vi "JTMonitor.vi"() -> ()   [LabVIEW 2016]
uses:
  Global/Global Variables/Data_Display_global.vi
panel:
  out "P5":dbl format="%#_13g"
  out "P3":dbl format="%#_13g"
  out "P2":dbl format="%#_13g"
  out "P1":dbl format="%#_13g"
  out "Comp":bool=TRUE
  out "FP":bool=TRUE
  out "V9":bool=TRUE
  out "V5":bool=TRUE
  out "V4":bool=TRUE
  out "V2":bool=TRUE
  out "V1":bool=TRUE
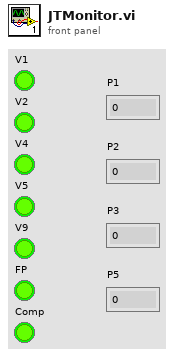
[diagram p1: front panel]
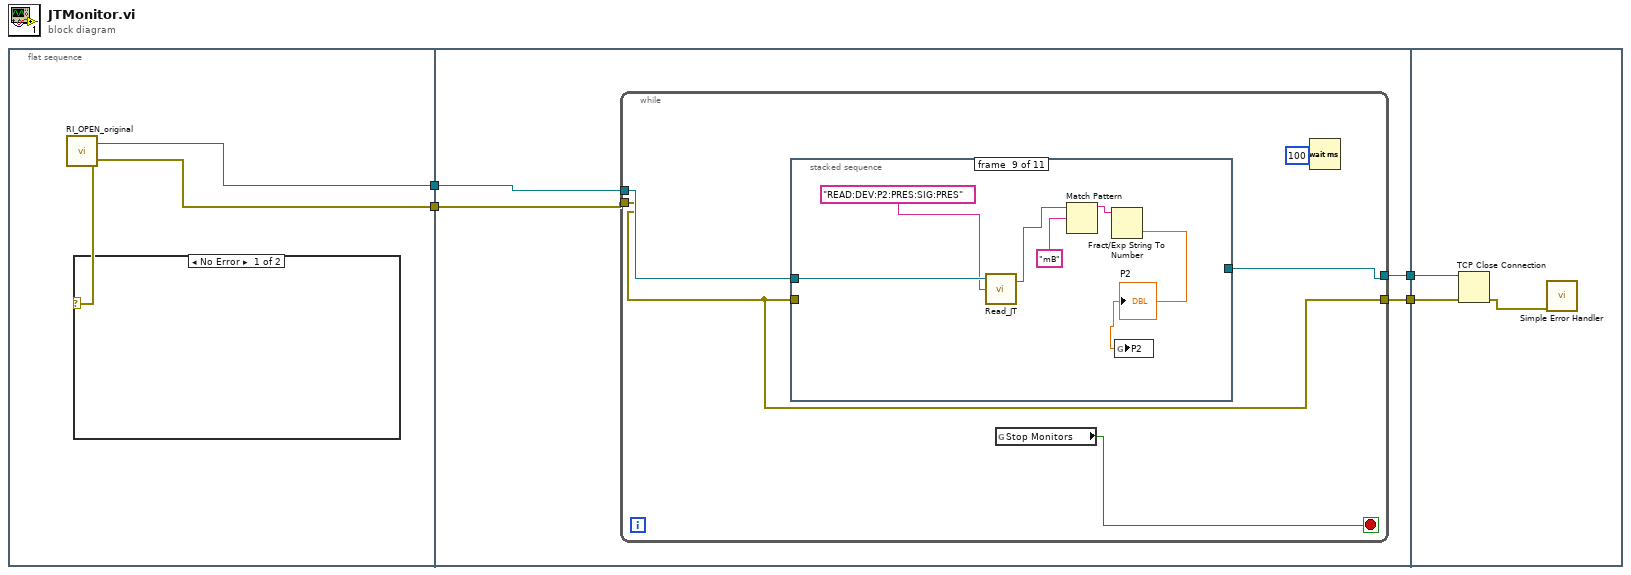
[diagram p0: block diagram]
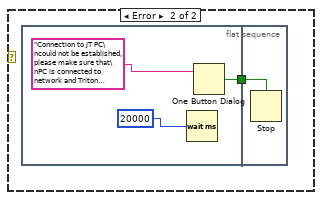
[diagram p2: hidden frame]
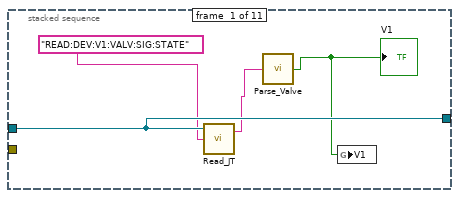
[diagram p3: hidden frame]
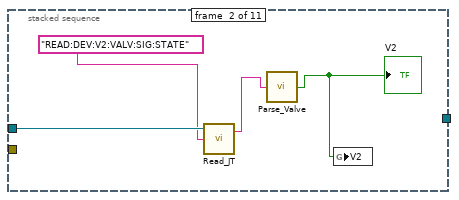
[diagram p4: hidden frame]
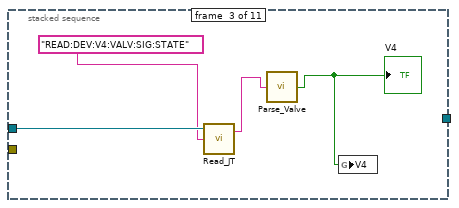
[diagram p5: hidden frame]
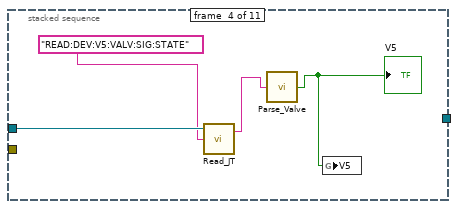
[diagram p6: hidden frame]
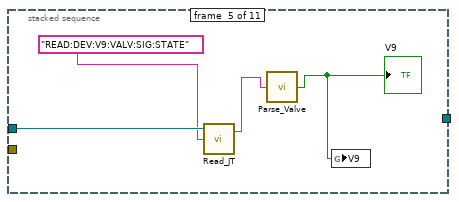
[diagram p7: hidden frame]
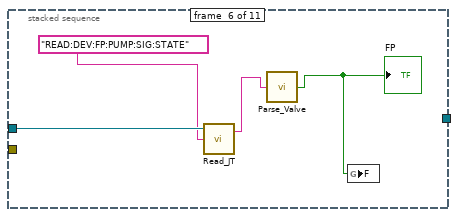
[diagram p8: hidden frame]
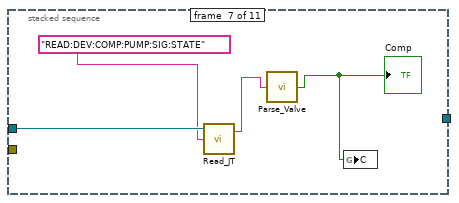
[diagram p9: hidden frame]
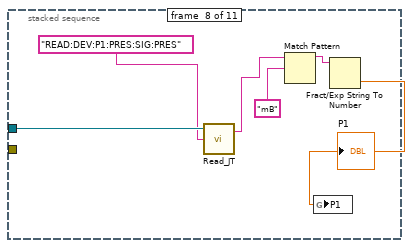
[diagram p10: hidden frame]
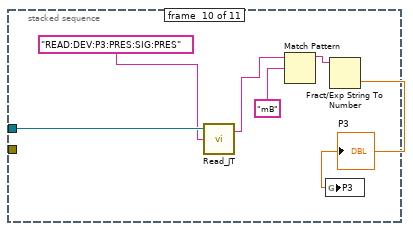
[diagram p11: hidden frame]
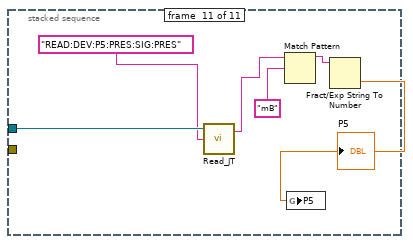
[diagram p12: hidden frame]
diagram:
  n1 = flat-sequence {
    tunnel: [w6] -> w2
    tunnel: [w5] -> w1
    tunnel: [w15] -> w4
    tunnel: [w14] -> w3
    tunnel: w2 -> [w13]
    tunnel: w1 -> [w12]
    tunnel: w4 -> [w74]
    tunnel: w3 -> [w73]
    frame #0 {
      n2 = call "RI_OPEN_original.vi"() -> ("error out"=w5:errorcluster, "connection ID"=w6:refnum<k5>)  [unwired: 3 in]
      n3 = case shown="No Error" w5 {
        frame No Error {
        }
        frame Error {
          n4 = flat-sequence {
            tunnel: [w8] -> w7
            tunnel: w7 -> [w11]
            frame #0 {
              n5 = Wait (ms)(milliseconds to wait=20000) -> ()  [unwired: 1 out]
              n6 = One Button Dialog(message="Connection to JT PC\ncould not be established, please make sure that\nPC is connected to network and Triton control software is running.\n\nThe JT monitor will be restarted in 20 seconds if the status monitor is not stopped meanwhile") -> (true=w8:bool)  [unwired: 1 in]
            }
            frame #1 {
              n7 = Stop(stop? (T)=w11) -> ()
            }
          }
        }
      }
    }
    frame #1 {
      n8 = while {
        tunnel: w13 -> [w19]
        tunnel: w12 -> [w17]
        tunnel: [w18] -> w15
        tunnel: [w17] -> w14
        stop <- w20 stop-if-true
        n9 = stacked-sequence {
          tunnel: w19 -> [w24 w28 w32 w36 w40 w44 w48 w54 w60 w66 w72]
          tunnel: [w24 _ _ _ _ _ _ _ _ _ _] -> w18
          tunnel: w17 -> [_ _ _ _ _ _ _ _ _ _ _]
          frame #0 {
            n10 = call "Read_JT.vi"("Write"="READ:DEV:V1:VALV:SIG:STATE", "connection ID"=w24) -> ("Read"=w22:string)  [unwired: 1 in, 1 out]
            n11 = call "Parse_Valve.vi"("Valve"=w22) -> ("Status"=w21:bool)
            "V1" <- w21
            n12 = global write "Data_Display_global.vi" "V1"(w21) -> ()
          }
          frame #1 {
            n13 = call "Read_JT.vi"("Write"="READ:DEV:V2:VALV:SIG:STATE", "connection ID"=w28) -> ("Read"=w26:string)  [unwired: 1 in, 1 out]
            n14 = call "Parse_Valve.vi"("Valve"=w26) -> ("Status"=w25:bool)
            "V2" <- w25
            n15 = global write "Data_Display_global.vi" "V2"(w25) -> ()
          }
          frame #2 {
            n16 = call "Read_JT.vi"("Write"="READ:DEV:V4:VALV:SIG:STATE", "connection ID"=w32) -> ("Read"=w30:string)  [unwired: 1 in, 1 out]
            n17 = call "Parse_Valve.vi"("Valve"=w30) -> ("Status"=w29:bool)
            "V4" <- w29
            n18 = global write "Data_Display_global.vi" "V4"(w29) -> ()
          }
          frame #3 {
            n19 = call "Read_JT.vi"("Write"="READ:DEV:V5:VALV:SIG:STATE", "connection ID"=w36) -> ("Read"=w34:string)  [unwired: 1 in, 1 out]
            n20 = call "Parse_Valve.vi"("Valve"=w34) -> ("Status"=w33:bool)
            "V5" <- w33
            n21 = global write "Data_Display_global.vi" "V5"(w33) -> ()
          }
          frame #4 {
            n22 = call "Read_JT.vi"("Write"="READ:DEV:V9:VALV:SIG:STATE", "connection ID"=w40) -> ("Read"=w38:string)  [unwired: 1 in, 1 out]
            n23 = call "Parse_Valve.vi"("Valve"=w38) -> ("Status"=w37:bool)
            "V9" <- w37
            n24 = global write "Data_Display_global.vi" "V9"(w37) -> ()
          }
          frame #5 {
            n25 = call "Read_JT.vi"("Write"="READ:DEV:FP:PUMP:SIG:STATE", "connection ID"=w44) -> ("Read"=w42:string)  [unwired: 1 in, 1 out]
            n26 = call "Parse_Valve.vi"("Valve"=w42) -> ("Status"=w41:bool)
            "FP" <- w41
            n27 = global write "Data_Display_global.vi" "F"(w41) -> ()
          }
          frame #6 {
            n28 = call "Read_JT.vi"("Write"="READ:DEV:COMP:PUMP:SIG:STATE", "connection ID"=w48) -> ("Read"=w46:string)  [unwired: 1 in, 1 out]
            n29 = call "Parse_Valve.vi"("Valve"=w46) -> ("Status"=w45:bool)
            "Comp" <- w45
            n30 = global write "Data_Display_global.vi" "C"(w45) -> ()
          }
          frame #7 {
            n31 = call "Read_JT.vi"("Write"="READ:DEV:P1:PRES:SIG:PRES", "connection ID"=w54) -> ("Read"=w52:string)  [unwired: 1 in, 1 out]
            n32 = Match Pattern(string=w52, regular expression="mB") -> (before substring=w50:string)  [unwired: 1 in, 3 out]
            n33 = Fract/Exp String To Number(string=w50) -> (number=w49:dbl)  [unwired: 3 in, 1 out]
            "P1" <- w49
            n34 = global write "Data_Display_global.vi" "P1"(w49) -> ()
          }
          frame #8 {
            n35 = call "Read_JT.vi"("Write"="READ:DEV:P2:PRES:SIG:PRES", "connection ID"=w60) -> ("Read"=w58:string)  [unwired: 1 in, 1 out]
            n36 = Match Pattern(string=w58, regular expression="mB") -> (before substring=w56:string)  [unwired: 1 in, 3 out]
            n37 = Fract/Exp String To Number(string=w56) -> (number=w55:dbl)  [unwired: 3 in, 1 out]
            "P2" <- w55
            n38 = global write "Data_Display_global.vi" "P2"(w55) -> ()
          }
          frame #9 {
            n39 = call "Read_JT.vi"("Write"="READ:DEV:P3:PRES:SIG:PRES", "connection ID"=w66) -> ("Read"=w64:string)  [unwired: 1 in, 1 out]
            n40 = Match Pattern(string=w64, regular expression="mB") -> (before substring=w62:string)  [unwired: 1 in, 3 out]
            n41 = Fract/Exp String To Number(string=w62) -> (number=w61:dbl)  [unwired: 3 in, 1 out]
            "P3" <- w61
            n42 = global write "Data_Display_global.vi" "P3"(w61) -> ()
          }
          frame #10 {
            n43 = call "Read_JT.vi"("Write"="READ:DEV:P5:PRES:SIG:PRES", "connection ID"=w72) -> ("Read"=w70:string)  [unwired: 1 in, 1 out]
            n44 = Match Pattern(string=w70, regular expression="mB") -> (before substring=w68:string)  [unwired: 1 in, 3 out]
            n45 = Fract/Exp String To Number(string=w68) -> (number=w67:dbl)  [unwired: 3 in, 1 out]
            "P5" <- w67
            n46 = global write "Data_Display_global.vi" "P5"(w67) -> ()
          }
        }
        n47 = global read "Data_Display_global.vi" "Stop Monitors"() -> (w20:bool)
        n48 = Wait (ms)(milliseconds to wait=100) -> ()  [unwired: 1 out]
      }
    }
    frame #2 {
      n49 = TCP Close Connection(connection ID=w74, error in (no error)=w73) -> (error out=w75:errorcluster)  [unwired: 1 in, 1 out]
      n50 = call <vilib>:"Simple Error Handler.vi"("error in (no error)"=w75) -> ()  [unwired: 4 in, 5 out]
    }
  }
